vi "Get Arc Velocity from Motors.vi"(6 "ccw caster motor velocity states":dbl[](array[numeric]), 7 "wheel indexes":i32[](array[numeric]), 8 "error in (no error)":errorcluster, 9 "ccw motor angle states (rad)":dbl[](array[numeric]), 10 "ccw motor velocity states":dbl[](array[numeric]), 11 "steering frame in":refnum<class "NI_Robotics_Steering Frame.lvclass">) -> (0 "error out":errorcluster, 2 "estimated arc velocity":T1={"turning radius"=1.0, "tangential velocity"=0.0, "angle from tangent (rad)"=0.0}, 3 "steering frame out":refnum<class "NI_Robotics_Steering Frame.lvclass">)   [LabVIEW 2017, in "NI_Robotics_Steering Frame.lvclass"]
doc: "Calculates the steering frame velocity or arc velocity required to best satisfy the velocity and angle of each motor. You must manually select the polymorphic instance to use."
uses:
  <vilib>/robotics/Steering/Steering Frame/NI_Robotics_Steering Frame.lvclass
  <vilib>/robotics/Steering/Steering Frame/Arc Velocity.ctl
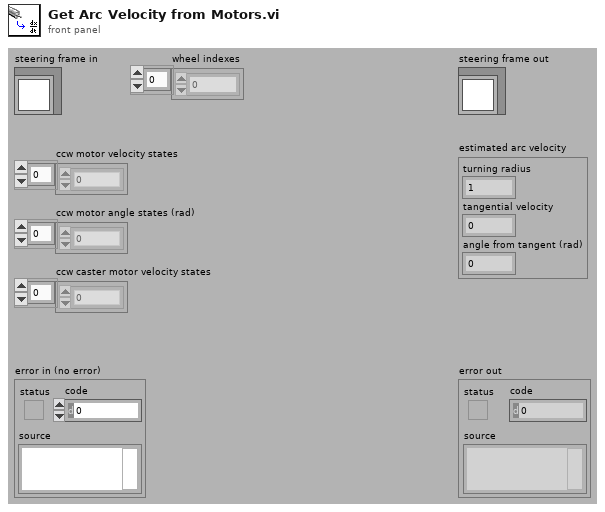
[diagram p1: front panel]
types:
  T1 = typedef "NI_Robotics_Steering Frame.lvclass/Arc Velocity.ctl" = cluster{"turning radius":dbl, "tangential velocity":dbl, "angle from tangent (rad)":dbl}
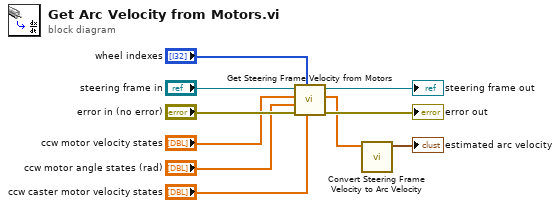
[diagram p0: block diagram]
diagram:
  n1 = call <vilib>:"Get Steering Frame Velocity from Motors.vi"("ccw caster motor velocity states"="ccw caster motor velocity states", "wheel indexes"="wheel indexes", "error in (no error)"="error in (no error)", "ccw motor angle states (rad)"="ccw motor angle states (rad)", "ccw motor velocity states"="ccw motor velocity states", "steering frame in"="steering frame in") -> ("error out"=→"error out":errorcluster, "estimated steering frame velocity"=w2:dbl[], "steering frame out"=→"steering frame out":refnum<class "NI_Robotics_Steering Frame.lvclass">)  [unwired: 3 in]
  n2 = call <vilib>:"Convert Steering Frame Velocity to Arc Velocity.vi"("steering frame velocity"=w2) -> ("arc velocity"=→"estimated arc velocity":T1)  [unwired: 10 in]
